vi "Test config files.vi"() -> ()   [LabVIEW 2015]
uses:
  HeliumMonitor/Sensor configuration.ctl
  HeliumMonitor/Channel type.ctl
  <vilib>/Utility/config.llb/NI_LVConfig.lvlib
panel:
  in  "configuration file path":path
  in  "Sensors":T1[](array[typedef])=[{"Name"="Ghz lab", "URL"="http:\\\\130.55.69.25", "Channels"=[{"type"=enum."Flow meter", "number"=6.0}]}, {"Name"="main bag", "URL"="http:\\\\130.55.69.22", "Channels"=[{"type"=enum."Flow meter", "number"=6.0}, {"type"=enum."Tank pressure", "number"=0.0}, {"type"=enum."Dewar level", "number"=1.0}]}, {"Name"="PPMS 20T", "URL"="http:\\\\130.55.69.42", "Channels"=[{"type"=enum."Flow meter", "number"=6.0}]}]
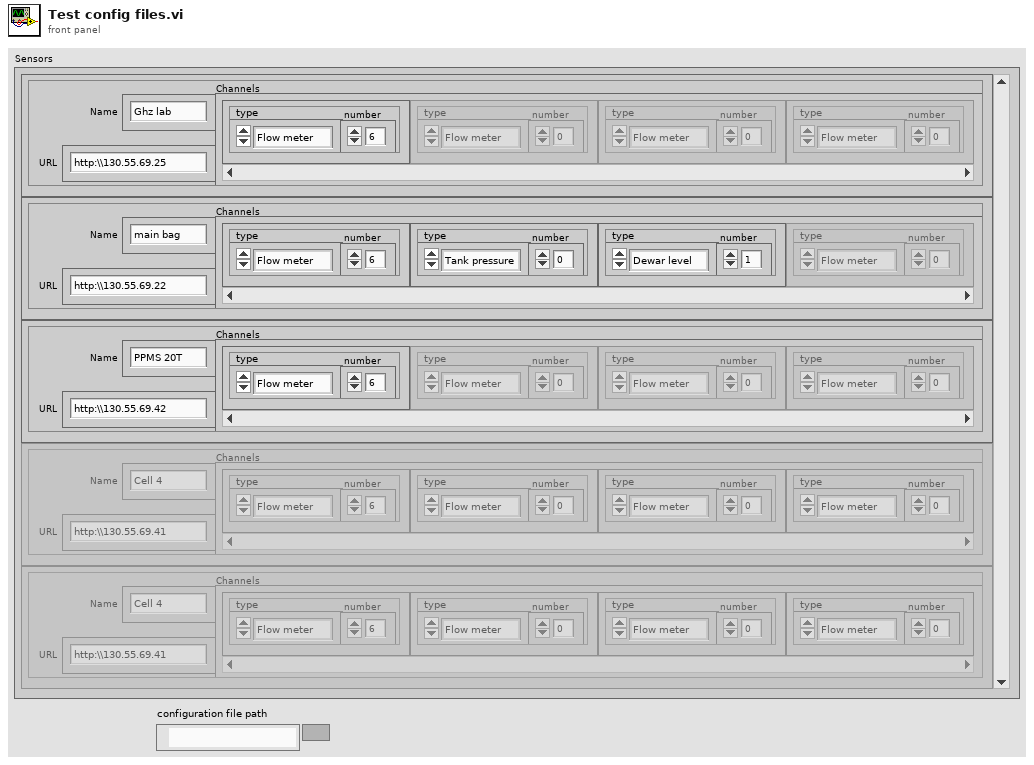
[diagram p1: front panel]
types:
  T1 = typedef "Sensor configuration.ctl" = cluster{"Name":string, "URL":string, "Channels":cluster{"type":T2, "number":dbl}[]}
  T2 = typedef "Channel type.ctl" = enum16{"Volts", "Flow meter", "Tank pressure", "Dewar level", "Raw ADC"}
  T3 = typedef "NI_LVConfig.lvlib/Config Data RefNum.ctl" = refnum<k1>
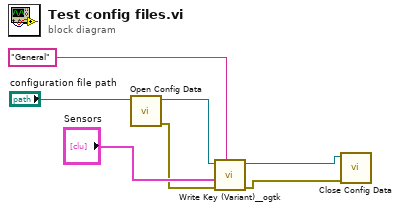
[diagram p0: block diagram]
diagram:
  n1 = call <vilib>:"Open Config Data.vi"("configuration file path"="configuration file path") -> ("error out"=w3:errorcluster, "refnum"=w6:T3)  [unwired: 8 in, 1 out]
  n2 = call <userlib>:"Write Key (Variant)__ogtk.vi"("section"="General", "error in (no error)"=w3, "key-value"="Sensors", "refnum"=w6) -> ("error out"=w4:errorcluster, "refnum out"=w7:T3)  [unwired: 6 in]
  n3 = call <vilib>:"Close Config Data.vi"("error in (no error)"=w4, "refnum"=w7) -> ()  [unwired: 8 in, 2 out]
